vi "DHTxx_Read.vi"(8 "error in (no error)":errorcluster) -> (0 "error out":errorcluster, 1 "f":sgl, 2 "c":sgl, 3 "h":sgl)   [LabVIEW 2014, in "QwaveSys RPi Training Library.lvlib"]
uses:
  <vilib>/Q-Wave Systems/QwaveSys RPi Package 2.0/Addons/QwaveSys RPi Training Library.lvlib
panel:
  out "return type":i32
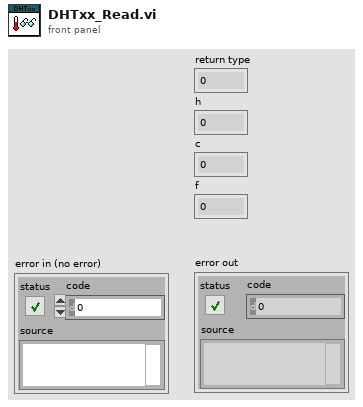
[diagram p1: front panel]
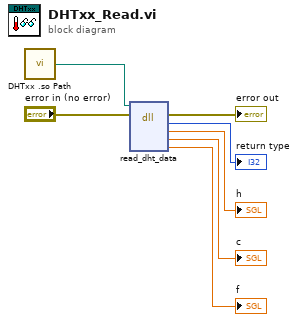
[diagram p0: block diagram]
diagram:
  n1 = call <vilib>:"DHTxx .so Path.vi"() -> ("DHTxx .so Path"=w5:path)  [unwired: 5 in]
  n2 = dll-call lib="libdht.so" fn="read_dht_data"(path in=w5, error in="error in (no error)") -> (error out=→"error out":errorcluster, "return type"=→"return type":i32, "h"=→"h":sgl, "c"=→"c":sgl, "f"=→"f":sgl)  [unwired: 4 in, 1 out]
